vi "get y.vi"(11 "Vector 2D in":refnum<class "Vector 2D.lvclass">) -> (3 "y":sgl)   [LabVIEW 2021, in "Vector 2D.lvclass"]
uses:
  Vector 2D.lvclass
  Vector 2D.lvclass/Vector 2D.ctl
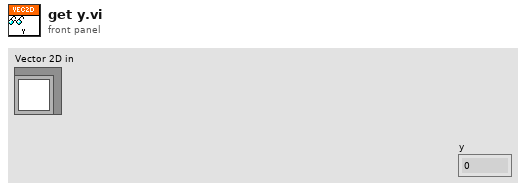
[diagram p1: front panel]
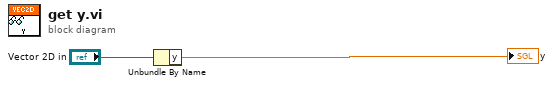
[diagram p0: block diagram]
diagram:
  n1 = Unbundle By Name("Vector 2D in") -> ("y"=→"y":sgl)
